vi "detectShape.vi"(1 "circle":i32, 2 "rectangle":i32, 3 "triangle":i32) -> (0 "String":string)   [LabVIEW 2023]
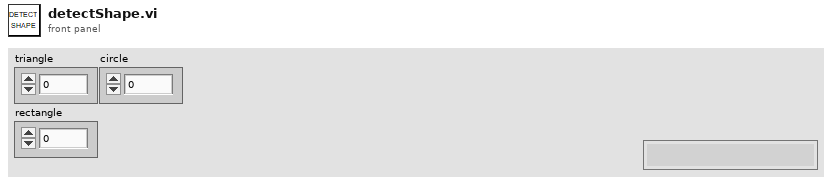
[diagram p1: front panel]
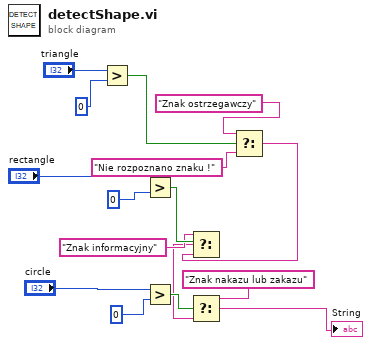
[diagram p0: block diagram]
diagram:
  n1 = Greater?(x="triangle", y=0) -> (0:w13:bool)
  n2 = Greater?(x="rectangle", y=0) -> (0:w11:bool)
  n3 = Greater?(x="circle", y=0) -> (0:w9:bool)
  n4 = Select(t="Znak ostrzegawczy", s=w13, f="Nie rozpoznano znaku !") -> (s? t:f=w5:string)
  n5 = Select(t="Znak informacyjny", s=w11, f=w5) -> (s? t:f=w4:string)
  n6 = Select(t="Znak nakazu lub zakazu", s=w9, f=w4) -> (s? t:f=→"String":string)
